vi "Data Buffer.vi"(5 "Datum in":dbl format="%.2f", 7 "task":enum16{"Init", "Write", "Read"}(ring)=enum."Write") -> (1 "Data out":dbl[](array[numeric]) format="%.2f")   [LabVIEW 2011]
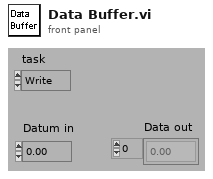
[diagram p1: front panel]
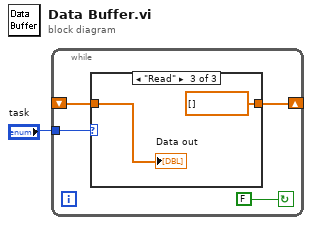
[diagram p0: block diagram]
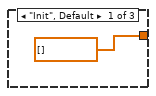
[diagram p2: hidden frame]
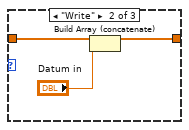
[diagram p3: hidden frame]
diagram:
  n1 = while {
    tunnel: "task" -> [w3]
    shift-left: _ -> [w5]
    shift-right: [w4] -> _
    stop <- FALSE continue-if-true
    n2 = case shown="\"Read\"" w3 {
      tunnel: w5 -> [_ w9 w10]
      tunnel: [dbl[] [] w8 dbl[] []] -> w4
      frame "Init", Default {
      }
      frame "Write" {
        n3 = Build Array (concatenate)(w9, "Datum in") -> (w8:dbl[])
      }
      frame "Read" {
        "Data out" <- w10
      }
    }
  }
